vi "Coord window-Estimate original Y coordinate.vi"(9 "Clicked coordinate":i32, 10 "Draw area width (pixels)":u32, 11 "FOV size (pixels)":i16) -> (2 "Coordinate (in um)":dbl)   [LabVIEW 2017]
uses:
  Global Variables/gl_UI Ctrl Refs.vi
  <vilib>/gmath/NI_Gmath.lvlib
panel:
  in  "Correction offset":i32=19
  in  "Draw area size correction":u32=5
  out "Location as fractional FOV index":dbl
  out "Relative pixel":i32
  out "Number of drawn FOVs (i.e. FOV visual range)":dbl
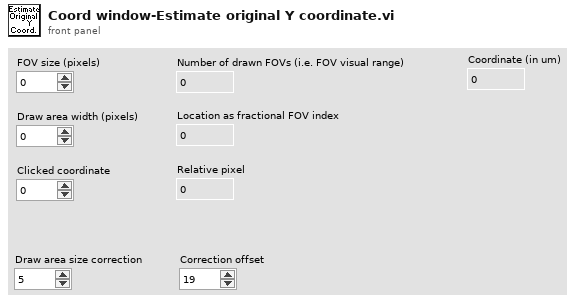
[diagram p1: front panel]
types:
  T1 = typedef "UI ctrl refs cluster.ctl" = cluster{"Top level VI path":path, "Top level VI ref":refnum<vi>, "User menu ref":refnum<k9>, "Sub Panel control":refnum<vi>, "Imaging Param Tab":refnum<vi>, "Occurrence-Start drivers":refnum<k4>, "Occurrence-Speed logging initialised":refnum<k4>, "Occurrence-XYZ stage initialised":refnum<k4>, "Exit button":refnum<vi>, "Status ind":refnum<vi>, "Set as origin":refnum<vi>, "Speed Logging":refnum<vi>, "Time Lapse":refnum<vi>, "Live Imaging":refnum<vi>, "AOL Z Stack":refnum<vi>, "Motor Z Stack":refnum<vi>, "Funct Acq button":refnum<vi>, "Hard Shutter":refnum<vi>, "Virtual Shutter":refnum<vi>, "Laser Power":refnum<vi>, "AOL Mode":refnum<vi>, "Frame Size":refnum<vi>, "Field of View":refnum<vi>, "Dwell Time":refnum<vi>, "Zoom":refnum<vi>, "AOL Z":refnum<vi>, "Objective":refnum<vi>, "Axis":refnum<vi>, "Paths & Names":refnum<vi>, "Experiment folder path (ind.)":refnum<vi>, "Last State (Ind.)":refnum<vi>, "Laser wavelength ind (nm)":refnum<vi>, "Averages":refnum<vi>, "Angle (degrees)":refnum<vi>, "X centre":refnum<vi>, "Y centre":refnum<vi>, "Plane Mode":refnum<vi>, "# Planes":refnum<vi>, "Z Start":refnum<vi>, "Z Stop":refnum<vi>, "Z Step":refnum<vi>, "PMT 1":refnum<vi>, "PMT 2":refnum<vi>, "Stage XYZ Position":refnum<vi>, "Pockels@Z Start":refnum<vi>, "Pockels@Z Stop":refnum<vi>, "Obtain Z Start":refnum<vi>, "Obtain Z Stop":refnum<vi>, "Live stim.trig.period":refnum<vi>, "Live stim.trig.enable":refnum<vi>, "Movement Correction":refnum<vi>, "Load Reference Image":refnum<vi>, "XY Stage Move":refnum<vi>, "MovCor Cluster":refnum<vi>, "RefDAQParam":refnum<vi>, "Funct. Acq. Pockels Modulation":refnum<vi>, "Background MovCor":refnum<vi>, "Ref Laser Power":refnum<vi>, "Enable Video Recording":refnum<vi>, "Video Record-Live Imaging":refnum<vi>, "Video Record-Funct acq":refnum<vi>, "Reference Source":refnum<vi>, "AOL Z-stack Chirps Ready (ind)":refnum<vi>, "Target time between mov.cor. ref triggers (ms)":refnum<vi>, "Funct. Acq. Ref frame save":refnum<vi>, "Tracking button":refnum<vi>, "Show ref plots window":refnum<vi>, "Center freq ind (nm)":refnum<vi>, "Pickup mode (ind)":refnum<vi>, "Logging queue (ind)":refnum<vi>, "Back aperture power (ind.)":refnum<vi>, "Power after objective (ind.)":refnum<vi>, "Switch user":refnum<vi>}
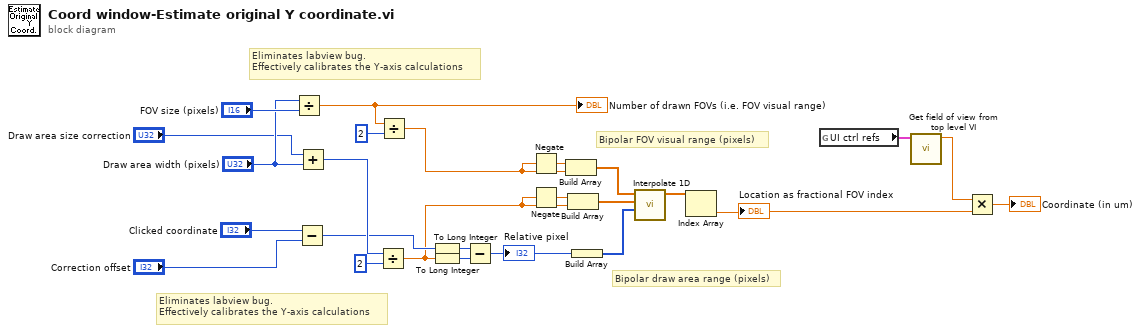
[diagram p0: block diagram]
diagram:
  # "Eliminates labview bug.\nEffectively calibrates the Y-axis calculations"
  # "Bipolar draw area range (pixels)"
  # "Bipolar FOV visual range (pixels)"
  # "Eliminates labview bug.\nEffectively calibrates the Y-axis calculations"
  n1 = Divide(x="Draw area width (pixels)", y="FOV size (pixels)") -> (x/y=w21:dbl)
  "Number of drawn FOVs (i.e. FOV visual range)" <- w21
  n2 = Subtract(x="Clicked coordinate", y="Correction offset") -> (x-y=w5:i32)
  n3 = Add(x="Draw area size correction", y="Draw area width (pixels)") -> (x+y=w8:u32)
  n4 = Divide(x=w8, y=u32 2) -> (x/y=w1:dbl)
  n5 = Divide(x=w21, y=u32 2) -> (x/y=w2:dbl)
  n6 = To Long Integer(number=w5) -> (32bit integer=w15:i32)
  n7 = To Long Integer(number=w1) -> (32bit integer=w16:i32)
  n8 = Subtract(x=w15, y=w16) -> (x-y=w18:i32)
  "Relative pixel" <- w18
  n9 = Negate(x=w2) -> (-x=w22:dbl)
  n10 = Negate(x=w1) -> (-x=w19:dbl)
  n11 = Build Array(w22, w2) -> (w11:dbl[])
  n12 = Build Array(w19, w1) -> (w12:dbl[])
  n13 = Build Array(w18) -> (w13:i32[])
  n14 = call <vilib>:"Interpolate 1D.vi"("xi"=w13, "X"=w12, "Y"=w11) -> ("yi"=w14:dbl[])  [unwired: 6 in, 2 out]
  n15 = Index Array(array=w14) -> (element=w3:dbl)  [unwired: 1 in]
  "Location as fractional FOV index" <- w3
  n16 = global read "gl_UI Ctrl Refs.vi" "UI ctrl refs"() -> (w25:T1)
  n17 = call "Get field of view from top level VI.vi"("UI ctrl refs"=w25) -> ("Field of view (um)"=w10:sgl)  [unwired: 10 in]
  n18 = Multiply(x=w10, y=w3) -> (x*y=→"Coordinate (in um)":dbl)
